vi "add ROI module.vi"(5 "校准步数":i32=40, 6 "参考球？":bool, 7 "ROI size":T8={"Left"=100, "Top"=100, "Right"=200, "Bottom"=200, "Rotation"=0.0} {"Rotation" min=-90.0 max=90.0 step=1.0 format="%.2f"; "Left" scale=0.0..1024.0; "Right" scale=0.0..1024.0}, 8 "error in (no error)":errorcluster caption="错误输入（无错误）", 10 "image control in":T1={"beads track"=[], "Public"={"标题名"="", "文件路径"=path "", "通道名"=[], "ROI Descriptor out"={"Global Rectangle"=[], "Contours"=[]}, "cali end"=0.0, "array piezo"=[], "LUT_R"=[], " ROI descriptors "=[{"Global Rectangle"=[0, 0, 0, 0], "Contours"=[{"ID"=enum."External", "Type"=12, "Coordinates"=[0, 0, 0, 0, 0]}]}, {"Global Rectangle"=[26, 104, 126, 204], "Contours"=[{"ID"=enum."External", "Type"=12, "Coordinates"=[26, 104, 126, 204, 0]}]}, {"Global Rectangle"=[99, 99, 201, 201], "Contours"=[{"ID"=enum."External", "Type"=12, "Coordinates"=[200, 200, 100, 100, 0]}]}], "tdms ref"=refnum, "分子长度(um)"=0.0, "ROI num"=0, "ROI size num"=[], "测量模式"=enum."force clamp"}, "beads info"=[]} {"Public"."ROI descriptors"."Contours"."Type" items=["No Selection", "Point", "Line", "Rectangle", "Oval", "Polygon", "Freehand Region", "Annulus", "Unused2", "Unused3", "Broken Line", "Freehand Line", "Rotated Rectangle"]; "Public"."ROI Descriptor out"."Contours"."Type" items=["No Selection", "Point", "Line", "Rectangle", "Oval", "Polygon", "Freehand Region", "Annulus", "Unused2", "Unused3", "Broken Line", "Freehand Line", "Rotated Rectangle"]; "beads track"."centroid"."Y Centroid" format="%.2f"; "beads track"."centroid"."X Centroid" format="%.2f"; "beads track"."ROI Des out"."Contours"."Type" items=["No Selection", "Point", "Line", "Rectangle", "Oval", "Polygon", "Freehand Region", "Annulus", "Unused2", "Unused3", "Broken Line", "Freehand Line", "Rotated Rectangle"]}, 11 "sample(quar)":i32) -> (0 "error out":errorcluster caption="错误输出", 1 "ROI Descriptor out":T3 {"Contours"."Type" items=["No Selection", "Point", "Line", "Rectangle", "Oval", "Polygon", "Freehand Region", "Annulus", "Unused2", "Unused3", "Broken Line", "Freehand Line", "Rotated Rectangle"]}, 2 "image control out":T1={"beads track"=[], "Public"={"标题名"="", "文件路径"=path "", "通道名"=[], "ROI Descriptor out"={"Global Rectangle"=[], "Contours"=[]}, "cali end"=0.0, "array piezo"=[], "LUT_R"=[], " ROI descriptors "=[{"Global Rectangle"=[0, 0, 0, 0], "Contours"=[{"ID"=enum."External", "Type"=12, "Coordinates"=[0, 0, 0, 0, 0]}]}, {"Global Rectangle"=[26, 104, 126, 204], "Contours"=[{"ID"=enum."External", "Type"=12, "Coordinates"=[26, 104, 126, 204, 0]}]}, {"Global Rectangle"=[99, 99, 201, 201], "Contours"=[{"ID"=enum."External", "Type"=12, "Coordinates"=[200, 200, 100, 100, 0]}]}], "tdms ref"=refnum, "分子长度(um)"=0.0, "ROI num"=0, "ROI size num"=[], "测量模式"=enum."force clamp"}, "beads info"=[]} {"Public"."ROI descriptors"."Contours"."Type" items=["No Selection", "Point", "Line", "Rectangle", "Oval", "Polygon", "Freehand Region", "Annulus", "Unused2", "Unused3", "Broken Line", "Freehand Line", "Rotated Rectangle"]; "Public"."ROI Descriptor out"."Contours"."Type" items=["No Selection", "Point", "Line", "Rectangle", "Oval", "Polygon", "Freehand Region", "Annulus", "Unused2", "Unused3", "Broken Line", "Freehand Line", "Rotated Rectangle"]; "beads track"."centroid"."Y Centroid" format="%.2f"; "beads track"."centroid"."X Centroid" format="%.2f"; "beads track"."ROI Des out"."Contours"."Type" items=["No Selection", "Point", "Line", "Rectangle", "Oval", "Polygon", "Freehand Region", "Annulus", "Unused2", "Unused3", "Broken Line", "Freehand Line", "Rotated Rectangle"]})   [LabVIEW 2017]
doc: "本VI是在监测窗口中增加一个ROI 框的功能集成VI。"
uses:
  ROI info.ctl
  control/Bead track.ctl
  control/beads public.ctl
  control/record mode.ctl
  control/bead info.ctl
  <vilib>/vision/Image Controls.llb/IMAQ Image.ctl
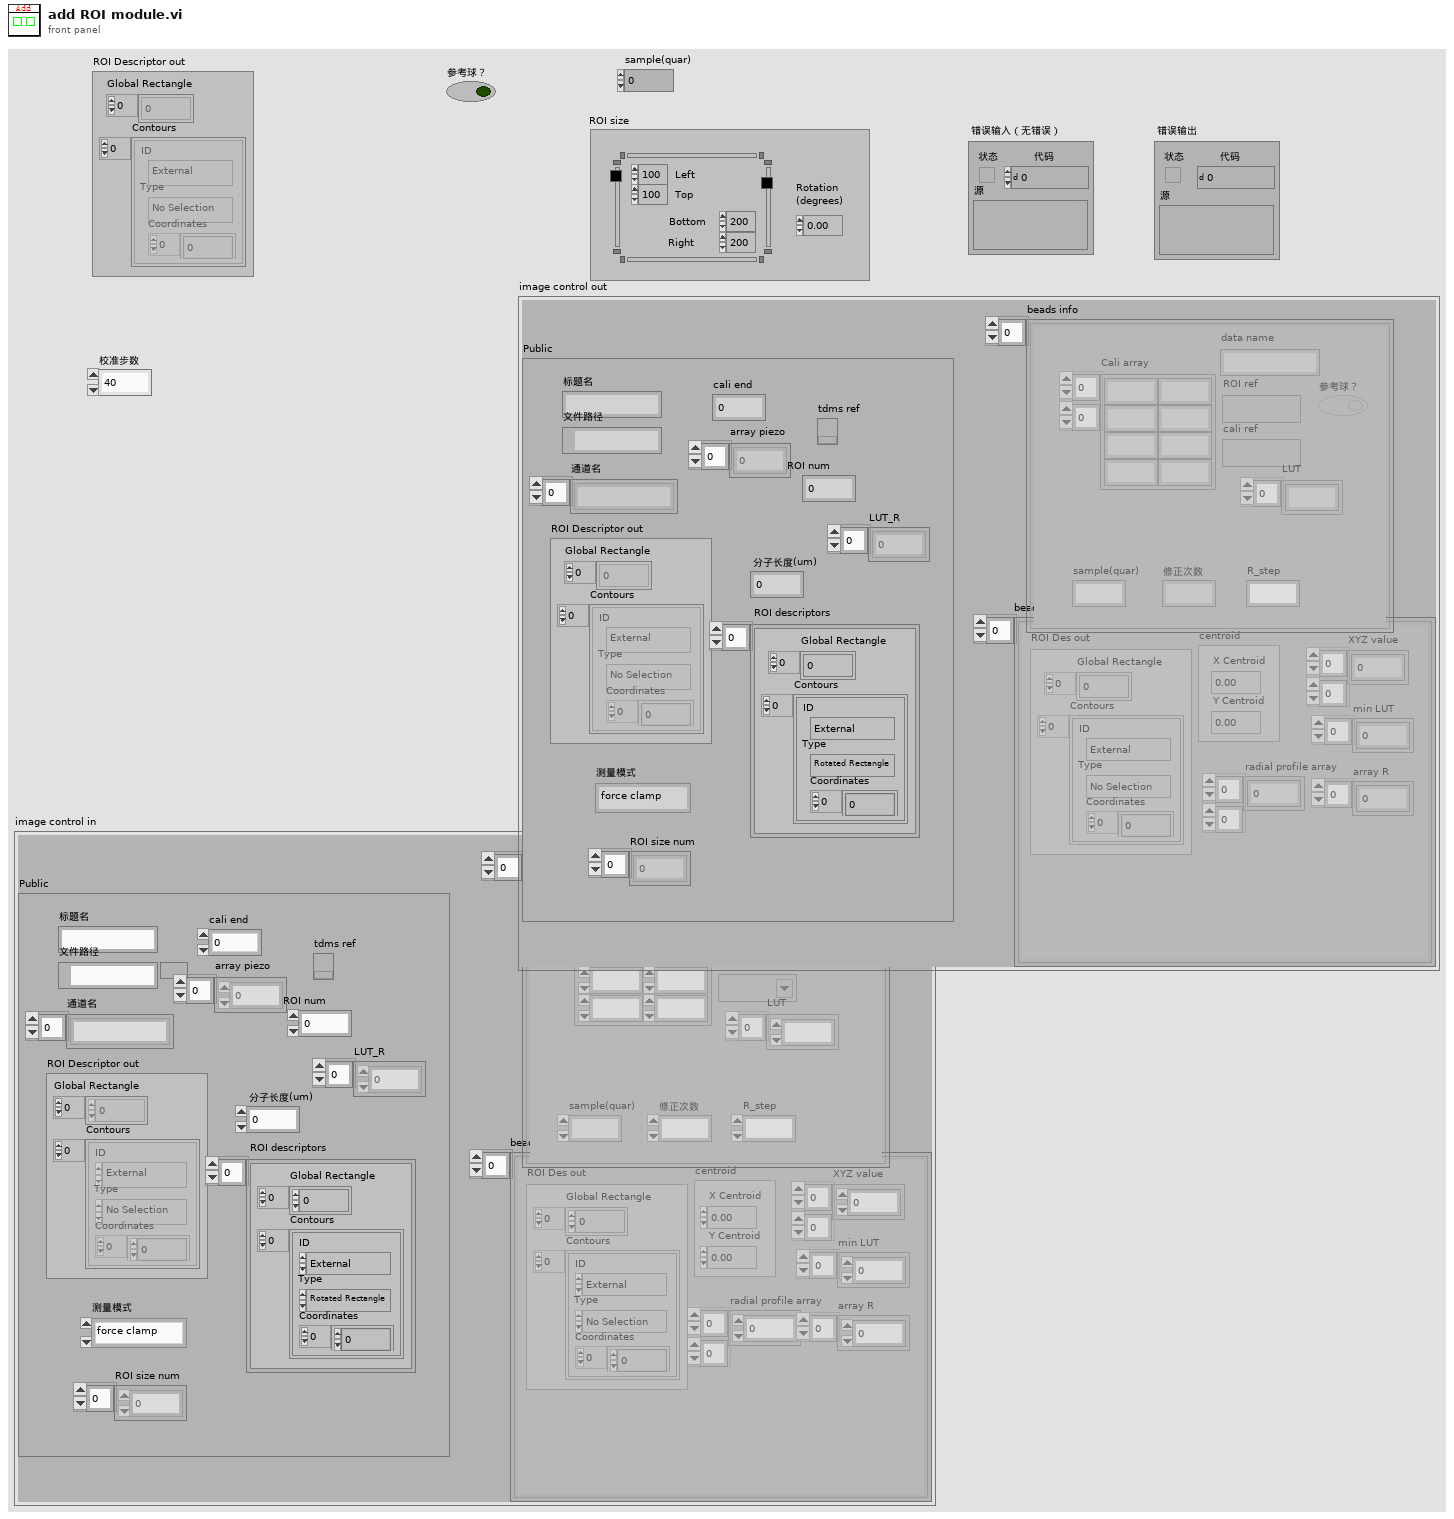
[diagram p1: front panel]
types:
  T1 = typedef "ROI info.ctl" = cluster{"beads track":T2[], "Public":T4, "beads info":T6[]}
  T2 = typedef "Bead track.ctl" = cluster{"XYZ value":dbl[][], "radial profile array":dbl[][], "min LUT":dbl[], "ROI Des out":T3, "array R":dbl[], "centroid":cluster{"X Centroid":sgl, "Y Centroid":sgl}}
  T3 = typedef "ROI Descriptor" = cluster{"Global Rectangle":i32[], "Contours":cluster{"ID":enum32{"External", "Internal"}, "Type":u32, "Coordinates":i32[]}[]}
  T4 = typedef "beads public.ctl" = cluster{"标题名":string, "文件路径":path, "通道名":string[], "ROI Descriptor out":T3, "cali end":dbl, "array piezo":dbl[], "LUT_R":dbl[], " ROI descriptors ":T3[], "tdms ref":refnum<k34>, "分子长度(um)":dbl, "ROI num":i32, "ROI size num":i32[], "测量模式":T5}
  T5 = typedef "record mode.ctl" = enum16{"force ramp", "force clamp", "user-defined", "force-mixed"}
  T6 = typedef "bead info.ctl" = cluster{"data name":string, "ROI ref":T7, "cali ref":T7, "参考球？":bool, "LUT":dbl[], "Cali array":dbl[][], "修正次数":i32, "R_step":dbl, "sample(quar)":i32}
  T7 = typedef "IMAQ Image.ctl" = refnum<image>
  T8 = typedef "IMAQ Rectangle" = cluster{"Left":i32, "Top":i32, "Right":i32, "Bottom":i32, "Rotation":dbl}
  T9 = typedef "Image Type" = u32
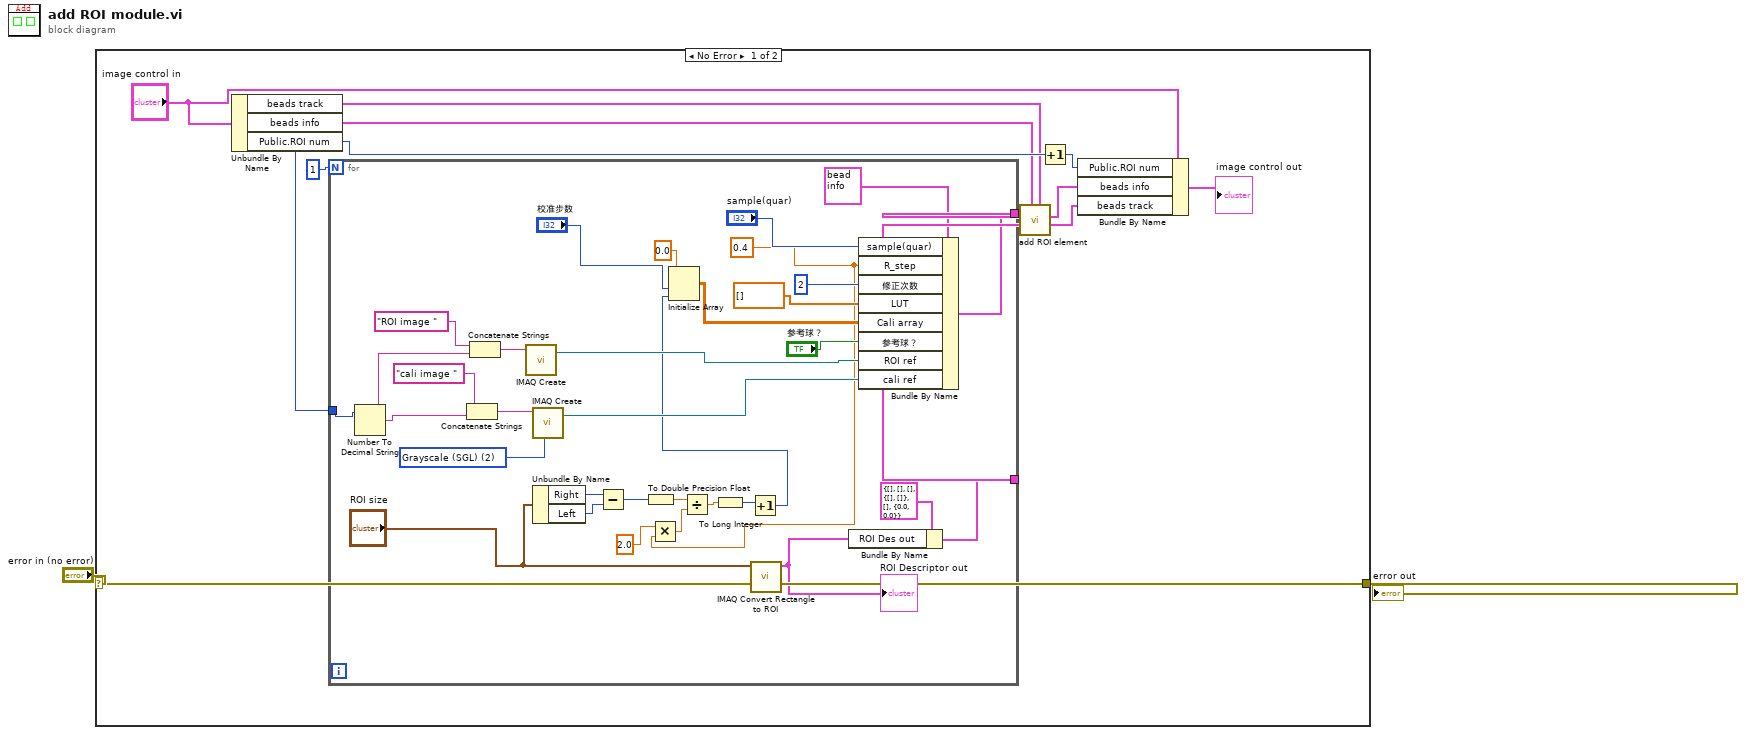
[diagram p0: block diagram]
diagram:
  n1 = case shown="No Error" "error in (no error)" {
    selector: "error in (no error)" -> [w14 w47]
    tunnel: [w14 w47] -> w1
    frame No Error {
      n2 = Unbundle By Name("image control in") -> ("beads track"=w7:T2[], "beads info"=w6:T6[], "Public.ROI num"=w11:i32)
      n3 = for "For循环" {
        N: 1 -> [_]
        tunnel: w11 -> [w28]
        tunnel: [w32] -> w9
        tunnel: [w31] -> w8
        w17 = 0.4 ("R_step")
        w42 = T9 2 items=["Grayscale (U8)", "Grayscale (I16)", "Grayscale (SGL)", "Complex (CSG)", "RGB (U32)", "HSL (U32)", "RGB (U64)", "Grayscale (U16)"] ("Image Type")
        n4 = Number To Decimal String(number=w28) -> (decimal integer string=w27:string)  [unwired: 1 in]
        n5 = Concatenate Strings("cali image " ("Image Name"), w27) -> (w43:string)
        n6 = Concatenate Strings("ROI image " ("Image Name"), w27) -> (w45:string)
        n7 = call "IMAQ Create"("Image Name"=w45) -> ("New Image"=w38:T7)  [unwired: 4 in, 1 out]
        n8 = call "IMAQ Create"("Image Name"=w43, "Image Type"=w42) -> ("New Image"=w37:T7)  [unwired: 3 in, 1 out]
        n9 = Unbundle By Name("ROI size") -> ("Right"=w24:i32, "Left"=w23:i32)
        n10 = Subtract(x=w24, y=w23) -> (x-y=w22:i32)
        n11 = To Double Precision Float(number=w22) -> (double precision float=w21:dbl)
        n12 = Multiply(x=2.0, y=w17) -> (x*y=w15:dbl)
        n13 = Divide(x=w21, y=w15) -> (x/y=w20:dbl)
        n14 = To Long Integer(number=w20) -> (32bit integer=w19:i32)
        n15 = Increment(x=w19) -> (x+1=w18:i32)
        n16 = Initialize Array(0.0 ("元素"), "校准步数", w18) -> (w39:dbl[][])
        n17 = call "IMAQ Convert Rectangle to ROI"("Rectangle"="ROI size") -> ("ROI Descriptor"=w33:T3)  [unwired: 8 in, 1 out]
        "ROI Descriptor out" <- w33
        n18 = Bundle By Name(cluster=T2 {"XYZ value"=[], "radial profile array"=[], "min LUT"=[], "ROI Des out"={"Global Rectangle"=[], "Contours"=[]}, "array R"=[], "centroid"={"X Centroid"=0.0, "Y Centroid"=0.0}} ("tracking"), "ROI Des out"=w33) -> (w31:T2)
        n19 = Bundle By Name(cluster=T6 {"data name"="", "ROI ref"=refnum, "cali ref"=refnum, "参考球？"=FALSE, "LUT"=[], "Cali array"=[], "修正次数"=0, "R_step"=0.0, "sample(quar)"=0} ("info"), "sample(quar)"="sample(quar)", "R_step"=w17, "修正次数"=2, "LUT"=dbl[] [], "Cali array"=w39, "参考球？"="参考球？", "ROI ref"=w38, "cali ref"=w37) -> (w32:T6)
      }
      n20 = call "add ROI element.vi"("beads track"=w7, "beads info"=w6, "tracking"=w8, "info"=w9) -> ("new track"=w4:T2[], "new info"=w5:T6[])  [unwired: 6 in]
      n21 = Increment(x=w11) -> (x+1=w10:i32)
      n22 = Bundle By Name(cluster="image control in", "Public.ROI num"=w10, "beads info"=w5, "beads track"=w4) -> (→"image control out":T1)
    }
    frame Error {
    }
  }
  "error out" <- w1
